vi "SimulatorHelperGetRobotsID.vi"(8 "error in (no error)":errorcluster, 11 "Enviroment":path) -> (0 "error out":errorcluster, 3 "Robots":string[](array[string]))   [LabVIEW 2015]
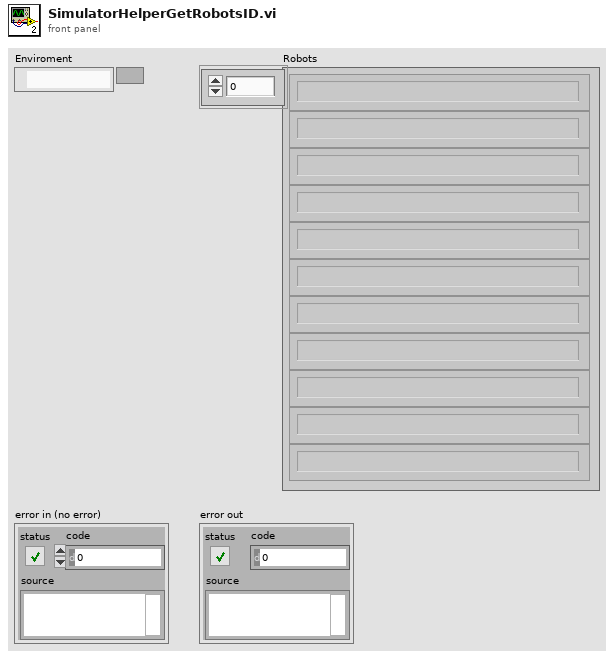
[diagram p1: front panel]
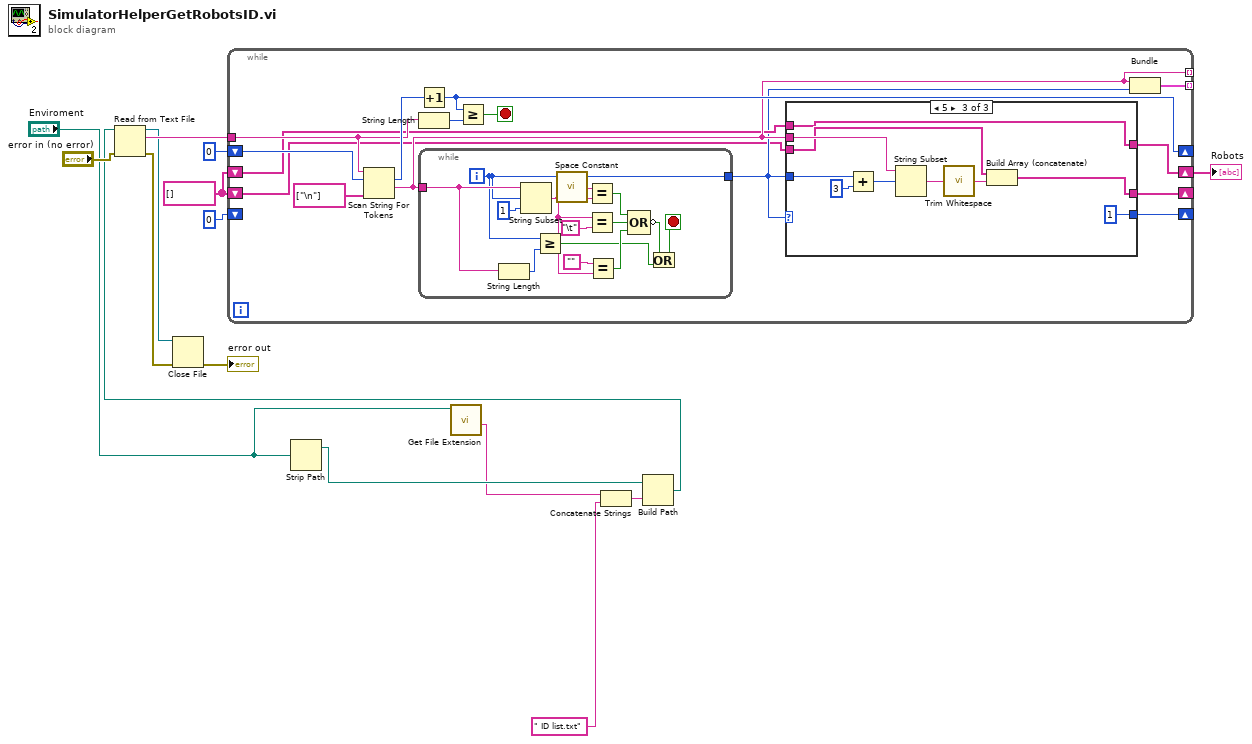
[diagram p0: block diagram]
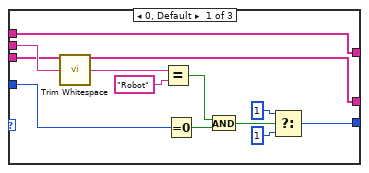
[diagram p2: hidden frame]
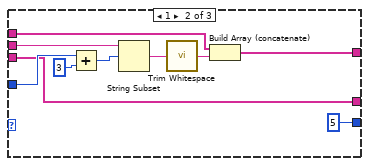
[diagram p3: hidden frame]
diagram:
  w14 = string[] []
  n1 = Strip Path(path="Enviroment") -> (stripped path=w3:path)  [unwired: 1 out]
  n2 = call <vilib>:"Get File Extension.vi"("file"="Enviroment") -> ("filename without extension"=w2:string)  [unwired: 6 in, 4 out]
  n3 = Concatenate Strings(w2, " ID list.txt" ("string")) -> (w5:string)
  n4 = Build Path(base path=w3, name or relative path=w5) -> (appended path=w1:path)
  n5 = Read from Text File(file (use dialog)=w1, error in="error in (no error)") -> (refnum out=w7:refnum<file>, text=w10:string, error out=w8:errorcluster)  [unwired: 2 in, 1 out]
  n6 = Close File(refnum=w7, error in=w8) -> (error out=→"error out":errorcluster)  [unwired: 1 out]
  n7 = while {
    tunnel: w10 -> [w27]
    shift-right: [w25] -> _
    shift-left: 0 ("offset past token") -> [w28]
    tunnel: [w22] -> _ mode=indexing
    tunnel: [w23] -> _ mode=indexing
    shift-right: [w21] -> _
    shift-left: u32 0 ("offset past token") -> [_]
    shift-right: [w20] -> w13
    shift-left: w14 -> [w19]
    shift-right: [w16] -> _
    shift-left: w14 -> [w17]
    stop <- w24 stop-if-true
    n8 = Scan String For Tokens(6:string[] ["\n"] ("delimiters (\\s,\\t,\\r,\\n)"), 8:w28, 9:w27) -> (1:w22:string, 2:w29:i32)  [unwired: 3 in, 2 out]
    n9 = Increment(x=w29) -> (x+1=w25:i32)
    n10 = String Length(string=w27) -> (length=w26:i32)
    n11 = while {
      tunnel: w22 -> [w68]
      tunnel: [w65] -> w18
      i -> [w65]
      stop <- w63 stop-if-true
      n12 = String Length(string=w68) -> (length=w66:i32)
      n13 = String Subset(string=w68, offset (0)=w65, length (rest)=1 ("length (rest)")) -> (substring=w72:string)
      n14 = Greater Or Equal?(x=w65, y=w66) -> (x >= y?=w64:bool)
      n15 = call <vilib>:"Space Constant.vi"() -> ("String"=w76:string)
      n16 = Equal?(x=w76, y=w72) -> (x = y?=w71:bool)
      n17 = Equal?(x=w72, y="\t") -> (x = y?=w70:bool)
      n18 = Equal?(x="", y=w72) -> (x = y?=w69:bool)
      n19 = Compound Arithmetic op=OR(w71, w70, w69) -> (invert w67:bool)
      n20 = Or(x=w67, y=w64) -> (x .or. y?=w63:bool)
    }
    n21 = Greater Or Equal?(x=w25, y=w26) -> (x >= y?=w24:bool)
    n22 = case shown="5" w18 {
      tunnel: w18 -> [w42 w48 w53]
      tunnel: w22 -> [w41 w49 w57]
      tunnel: [w34 u32 5 ("f") u32 1 ("f")] -> w21
      tunnel: [w32 w51 w54] -> w20
      tunnel: w19 -> [w32 w50 w54]
      tunnel: w17 -> [w31 w43 w56]
      tunnel: [w31 w43 w55] -> w16
      frame 0, Default {
        n23 = call <vilib>:"Trim Whitespace.vi"("string"=w41) -> ("trimmed string"=w40:string)  [unwired: 1 in]
        n24 = Equal?(x=w40, y="Robot") -> (x = y?=w38:bool)
        n25 = Equal To 0?(x=w42) -> (x = 0?=w37:bool)
        n26 = And(x=w38, y=w37) -> (x .and. y?=w36:bool)
        n27 = Select(t=u32 1, s=w36, f=u32 1) -> (s? t:f=w34:u32)
      }
      frame 1 {
        n28 = Add(x=w48, y=3) -> (x+y=w47:i32)
        n29 = String Subset(string=w49, offset (0)=w47) -> (substring=w45:string)  [unwired: 1 in]
        n30 = call <vilib>:"Trim Whitespace.vi"("string"=w45) -> ("trimmed string"=w44:string)  [unwired: 1 in]
        n31 = Build Array (concatenate)(w50, w44) -> (w51:string[])
      }
      frame 5 {
        n32 = Add(x=w53, y=3) -> (x+y=w61:i32)
        n33 = String Subset(string=w57, offset (0)=w61) -> (substring=w59:string)  [unwired: 1 in]
        n34 = call <vilib>:"Trim Whitespace.vi"("string"=w59) -> ("trimmed string"=w58:string)  [unwired: 1 in]
        n35 = Build Array (concatenate)(w56, w58) -> (w55:string[])
      }
    }
    n36 = Bundle("token string"=w22, w18) -> (w23:cluster{"token string":string, i32})  [unwired: 1 in]
  }
  "Robots" <- w13
